vi "Semaphore Post.vi"(8 "error in (no error)":errorcluster, 11 "Semaphore in":T1) -> (0 "error out":errorcluster, 3 "Semaphore out":T1)   [LabVIEW 2013, in "POSIX Threads.lvlib" / "Semaphore.lvclass"]
doc: "Calls sem_post() on a semaphore referenced by the provided Semaphore object. Posting increases a sempahore's count by 1 which can be used to signal other processes currently using Semaphore Wait."
uses:
  Semaphore.lvclass
  Controls/reference.ctl
  POSIX Thread Object/POSIX Thread Object.lvclass/POSIX Thread Object.ctl
  POSIX Thread Object/Private VIs/libpthread path.vi
  POSIX Thread Object/Private VIs/get pthread error.vi
  <vilib>/NI/NI Linux RT Errno/VIs/Public/Get Errno Value for Calling Thread.vi
  POSIX Thread Object/POSIX Thread Object.lvclass
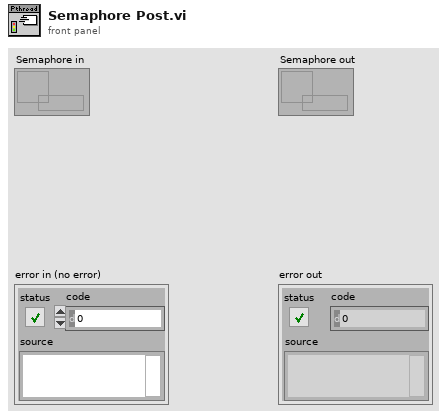
[diagram p1: front panel]
types:
  T1 = typedef "POSIX Threads.lvlib/Semaphore.lvclass/reference.ctl" = refnum<data-value>
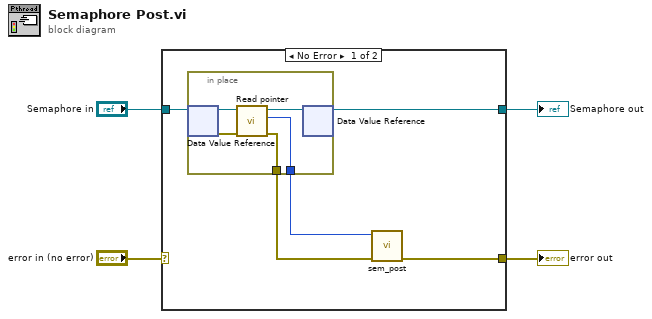
[diagram p0: block diagram]
diagram:
  n1 = case shown="No Error" "error in (no error)" {
    selector: "error in (no error)" -> [_ w15]
    tunnel: "Semaphore in" -> [w9 w16]
    tunnel: [w8 w16] -> w1
    tunnel: [w7 w15] -> w2
    frame No Error {
      n2 = in-place {
        in-place-border: [w11] -> w6
        in-place-border: [w10] -> w5
        n3 = in-place-dvr #1(w9) -> (w14:refnum<class "Semaphore.lvclass">, w13:errorcluster)
        n4 = call "Read pointer.vi"("error in (no error)"=w13, "POSIX Thread Object in"=w14) -> ("error out"=w11:errorcluster, "pointer"=w10:u64, "POSIX Thread Object out"=w12:refnum<class "Semaphore.lvclass">)  [unwired: 7 in]
        n5 = in-place-dvr #1(w12) -> (w8:T1)  [unwired: 1 out]
      }
      n6 = call "sem_post.vi"("error in (no error)"=w6, "sempahore ptr in"=w5) -> ("error out"=w7:errorcluster)  [unwired: 8 in, 1 out]
    }
    frame Error {
    }
  }
  "error out" <- w2
  "Semaphore out" <- w1
